vi "Get Driver Joystick State.vi"(8 "error in (no error)":errorcluster, 10 "Joystick State":T1, 11 "Driver in":refnum<class "Driver.lvclass">) -> (0 "error out":errorcluster, 3 "Driver out":refnum<class "Driver.lvclass">)   [LabVIEW 2014, in "Driver.lvlib" / "Driver.lvclass"]
uses:
  Driver.lvclass
  Joystick/Joystick Class/Joystick State.ctl
  Joystick/Joystick Class/Button State.ctl
  Joystick/Joystick Class/Axis State.ctl
  Joystick/Joystick Class/Joystick.lvclass
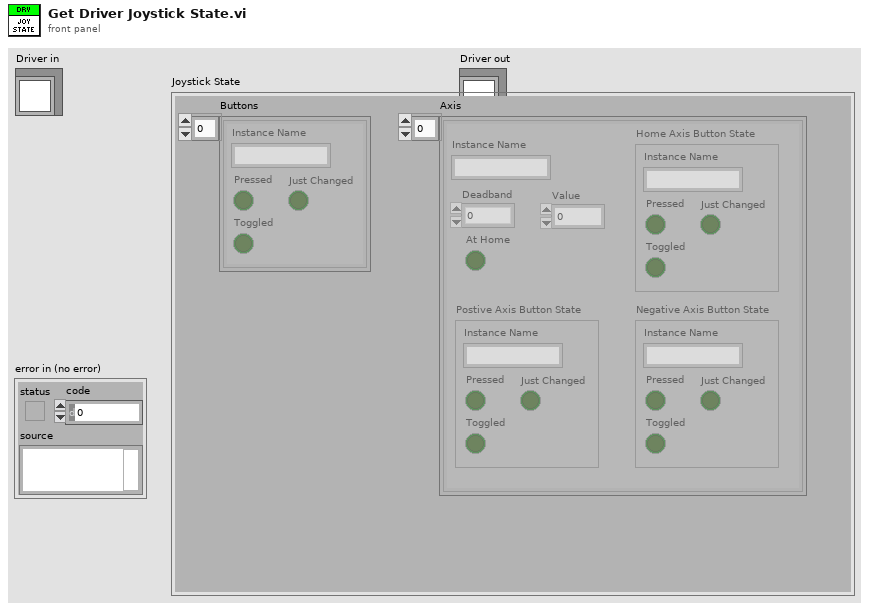
[diagram p1: front panel]
types:
  T1 = typedef "Joystick.lvlib/Joystick.lvclass/Joystick State.ctl" = cluster{"Buttons":T2[], "Axis":T3[]}
  T2 = typedef "Joystick.lvlib/Joystick.lvclass/Button State.ctl" = cluster{"Pressed":bool, "Instance Name":string, "Toggled":bool, "Just Changed":bool}
  T3 = typedef "Joystick.lvlib/Joystick.lvclass/Axis State.ctl" = cluster{"Instance Name":string, "Deadband":dbl, "Value":dbl, "At Home":bool, "Postive Axis Button State":T2, "Negative Axis Button State":T2, "Home Axis Button State":T2}
  T4 = enum16{"Critical", "Error", "Warning", "Informational", "Debug"}
  T5 = typedef "Driver.lvlib/Driver.lvclass/Driver State.ctl" = cluster{"Forward Joystick":dbl, "Rotate Right Joystick":dbl, "Slide Right Joystick":dbl, "Last Joystick State":cluster{"Buttons":T2[], "Axis":T3[]}}
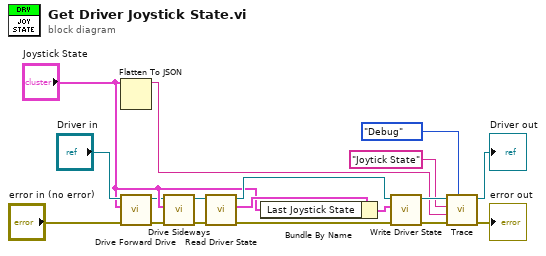
[diagram p0: block diagram]
diagram:
  n1 = Flatten To JSON(anything="Joystick State") -> (JSON string=w9:string)  [unwired: 2 in, 1 out]
  n2 = call-dynamic "Drive Forward Drive.vi"("error in (no error)"="error in (no error)", "Joystick State"="Joystick State", "Driver in"="Driver in") -> ("error out"=w5:errorcluster, "Driver out"=w8:refnum<class "Driver.lvclass">)  [unwired: 7 in]
  n3 = call-dynamic "Drive Sideways.vi"("error in (no error)"=w5, "Joystick State"="Joystick State", "Driver in"=w8) -> ("error out"=w4:errorcluster, "Driver out"=w7:refnum<class "Driver.lvclass">)  [unwired: 7 in]
  n4 = call-dynamic "Read Driver State.vi"("error in (no error)"=w4, "Driver in"=w7) -> ("error out"=w3:errorcluster, "Driver State"=w17:T5, "Driver out"=w18:refnum<class "Driver.lvclass">)  [unwired: 7 in]
  n5 = Bundle By Name(cluster=w17, "Last Joystick State"="Joystick State") -> (w16:T5)
  n6 = call-dynamic "Write Driver State.vi"("error in (no error)"=w3, "Driver State"=w16, "Driver in"=w18) -> ("error out"=w2:errorcluster, "Driver out"=w14:refnum<class "Driver.lvclass">)  [unwired: 7 in]
  n7 = call-dynamic "Trace.vi"("Trace Level"=T4."Debug", "error in (no error)"=w2, "System Message"=w9, "System Action"="Joytick State", "System Actor in"=w14) -> ("error out"=→"error out":errorcluster, "System Actor out"=→"Driver out":refnum<class "Driver.lvclass">)  [unwired: 5 in]
